vi "Group Filter Tree.vi"(8 "error in":errorcluster, 11 "Data in":string[][](array[string])=[["2020.12.05.", "0x710", "can", "rx", "6", "01 02 03 04 05 05", "", "", ""], ["", "", "", "", "", "", "fram1", "sign1", "10"], ["", "", "", "", "", "", "fram2", "sign2", "15"], ["2021.02.01.", "0x720", "can", "rx", "3", "01 02 03", "", "", ""], ["", "", "", "", "", "", "fram3", "sign3", "30"], ["", "", "", "", "", "", "fram4", "sign4", "5"], ["", "", "", "", "", "", "fram5", "sign5", "10"]]) -> (0 "error IO":errorcluster, 3 "Frame groups":T1(array[cluster]))   [LabVIEW 2025, in "CAN-LIN Raw Bus Capture UI.lvlib"]
uses:
  CAN-LIN Raw Bus Capture UI.lvlib
  <vilib>/Utility/error.llb/whitespace.ctl
  <vilib>/Utility/error.llb/Trim Whitespace One-Sided.vi
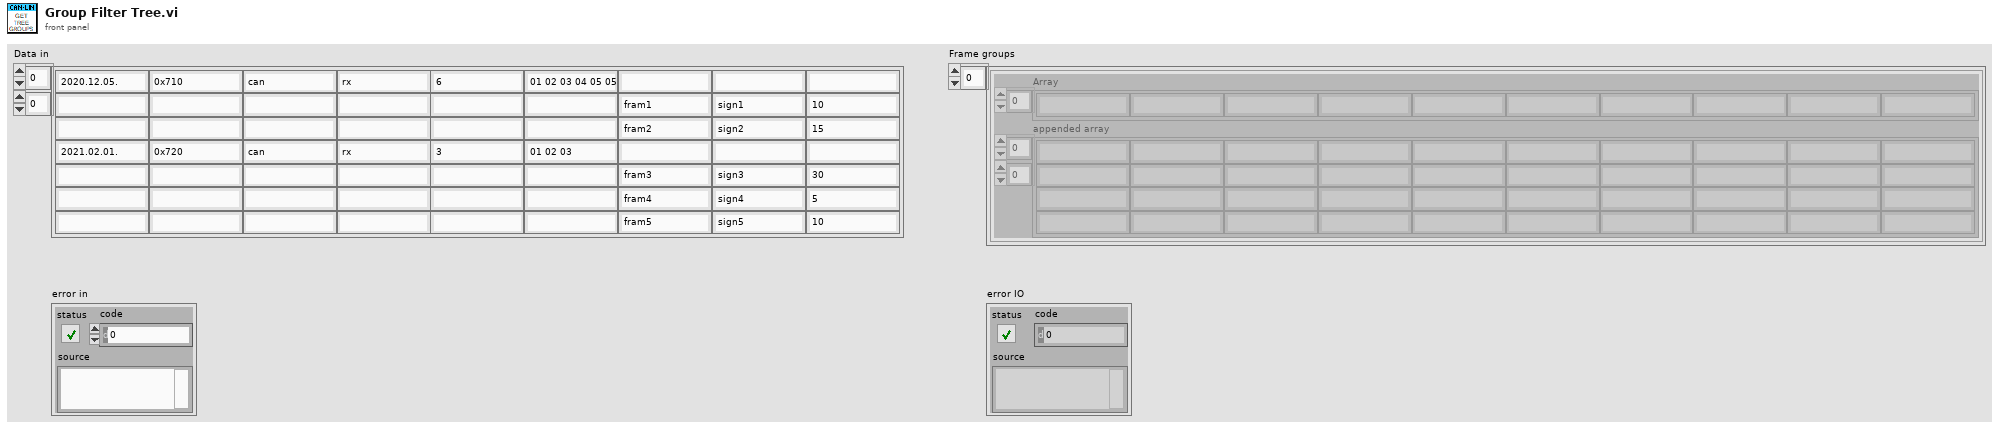
[diagram p1: front panel]
types:
  T1 = cluster{"Array":string[], "appended array":string[][]}[]
  T2 = cluster{"Root":string[], "Child rows":string[][]}[]
  T3 = typedef "whitespace.ctl" = u16
  T4 = cluster{"Array":string[], "appended array":string[][]}
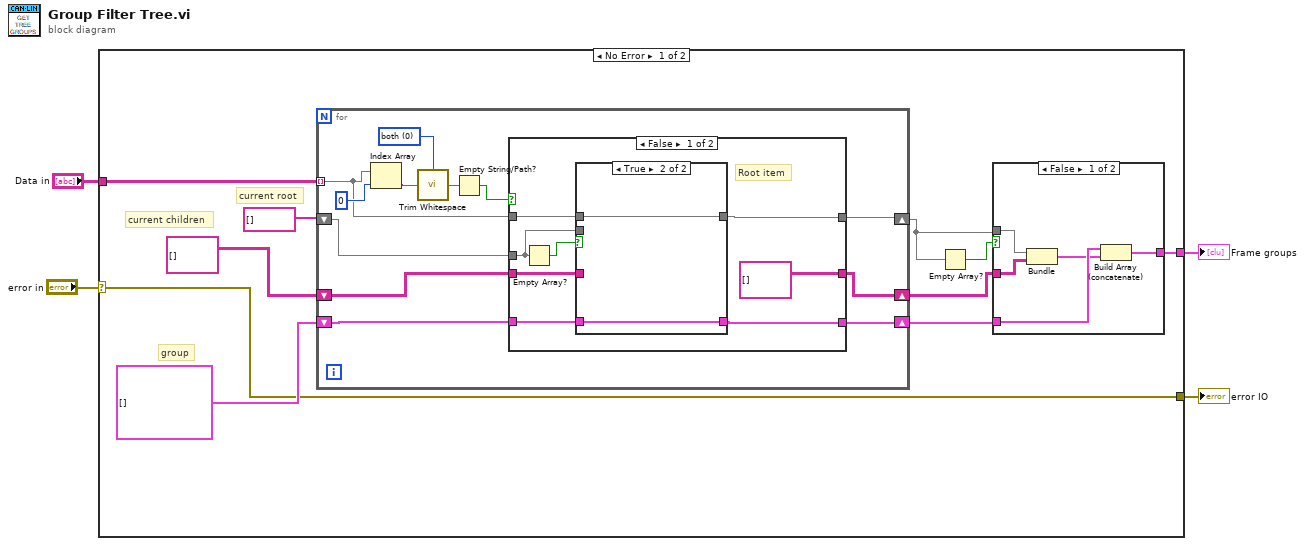
[diagram p0: block diagram]
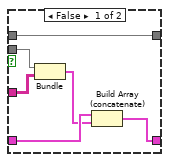
[diagram p2: hidden frame]
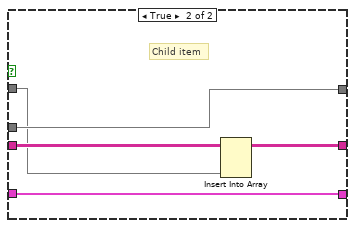
[diagram p3: hidden frame]
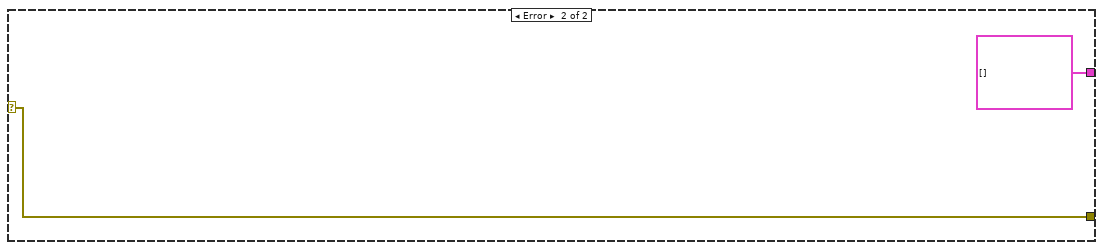
[diagram p5: hidden frame]
diagram:
  n1 = case shown="No Error" "error in" {
    selector: "error in" -> [w5 w55]
    tunnel: [w7 T2 []] -> w4
    tunnel: "Data in" -> [w6 _]
    tunnel: [w5 w55] -> w2
    frame No Error {
      # "group"
      # "current children"
      # "current root"
      n2 = for {
        tunnel: w6 -> [w19] mode=indexing
        shift-right: [w17] -> w10
        shift-left: string[] [] ("Array") -> [w21]
        shift-right: [w18] -> w9
        shift-left: string[][] [] ("appended array") -> [w20]
        shift-right: [w16] -> w8
        shift-left: T2 [] -> [w15]
        w24 = T3 0 items=["both", "start of string", "end of string"] ("location (both)")
        n3 = Index Array(array=w19, index=0) -> (element=w22:string)
        n4 = call <vilib>:"Trim Whitespace.vi"("string"=w22, "location (both)"=w24) -> ("trimmed string"=w25:string)
        n5 = Empty String/Path?(string/path=w25) -> (empty?=w23:bool)
        n6 = case shown="False" w23 {
          tunnel: w19 -> [w30 w45]
          tunnel: [w29 w47] -> w17
          tunnel: w21 -> [w32 w47]
          tunnel: w20 -> [w31 w46]
          tunnel: [string[][] [] ("appended array") w44] -> w18
          tunnel: [w28 w43] -> w16
          tunnel: w15 -> [w27 w43]
          frame False {
            # "Root item"
            n7 = Empty Array?(array=w32) -> (empty?=w33:bool)
            n8 = case shown="True" w33 {
              tunnel: w32 -> [w39 _]
              tunnel: w31 -> [w38 _]
              tunnel: w30 -> [w40 w42]
              tunnel: [w40 w42] -> w29
              tunnel: [w35 w41] -> w28
              tunnel: w27 -> [w37 w41]
              frame False {
                n9 = Bundle("Array"=w39, "appended array"=w38) -> (w36:T4)  [unwired: 1 in]
                n10 = Build Array (concatenate)(w37, w36) -> (w35:T1)
              }
              frame True {
              }
            }
          }
          frame True {
            # "Child item"
            n11 = Insert Into Array(array=w46, new element=w45) -> (w44:string[][])  [unwired: 2 in]
          }
        }
      }
      n12 = Empty Array?(array=w10) -> (empty?=w11:bool)
      n13 = case shown="False" w11 {
        tunnel: w10 -> [w52 _]
        tunnel: w9 -> [w51 _]
        tunnel: [w48 w53] -> w7
        tunnel: w8 -> [w50 w53]
        frame False {
          n14 = Bundle("Array"=w52, "appended array"=w51) -> (w49:T4)  [unwired: 1 in]
          n15 = Build Array (concatenate)(w50, w49) -> (w48:T1)
        }
        frame True {
        }
      }
    }
    frame Error {
    }
  }
  "Frame groups" <- w4
  "error IO" <- w2
